vi "Save.vi"(8 "error in (no error)":errorcluster, 10 "Path":path=path "", 11 "Plot ID In":T1 format="%x") -> (0 "error out":errorcluster, 3 "Plot ID Out":T1 format="%x")   [LabVIEW 2013, in "Advanced Plotting Toolkit.lvlib"]
doc: "Save the plot to disk. The format is determined by the file extension. Supported formats are PDF, PNG, BMP, TIFF, JPEG, and GIF."
uses:
  Advanced Plotting Toolkit.lvlib
  typedefs/PlotID.ctl
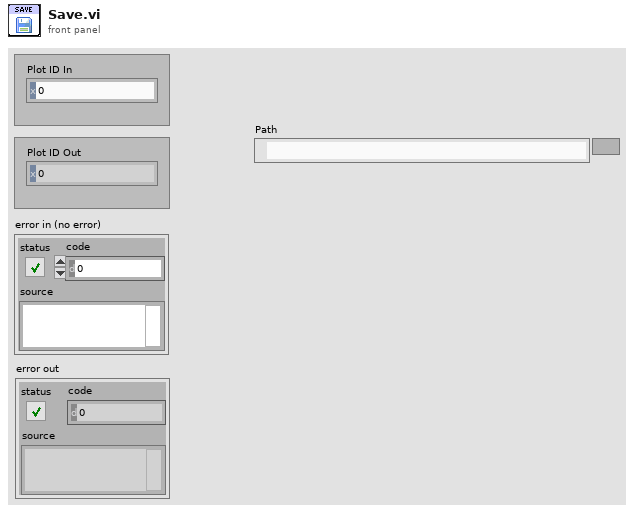
[diagram p1: front panel]
types:
  T1 = typedef "Advanced Plotting Toolkit.lvlib/PlotID.ctl" = i32
  T2 = typedef "Advanced Plotting Toolkit.lvlib/KeyValue.ctl" = cluster{"Key":string, "Value":string}
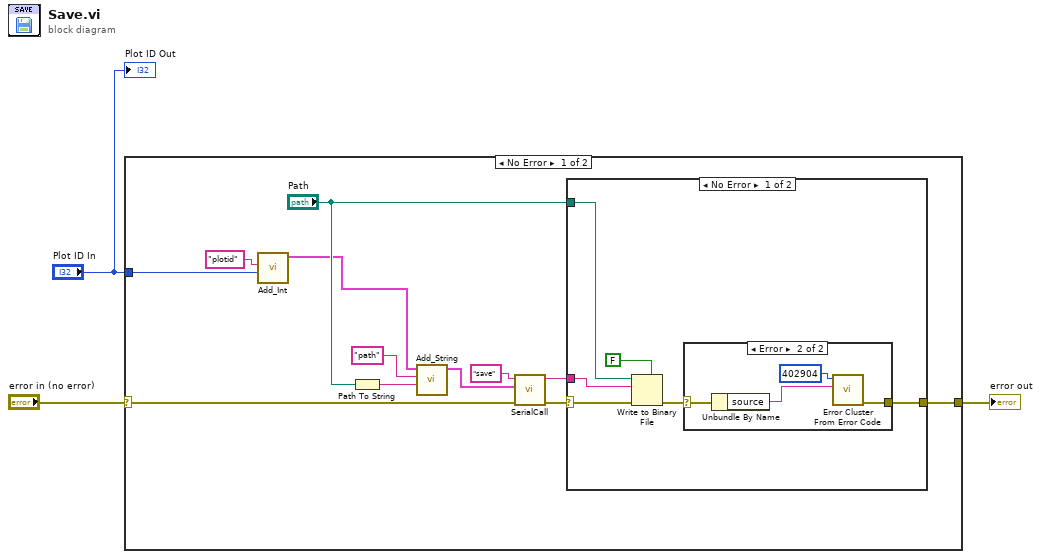
[diagram p0: block diagram]
diagram:
  n1 = case shown="No Error" "error in (no error)" {
    selector: "error in (no error)" -> [w11 w28]
    tunnel: "Plot ID In" -> [w10 _]
    tunnel: [w12 w28] -> w2
    frame No Error {
      n2 = call "Add_Int.vi"("Value"=w10, "Key"="plotid" ("Keyword")) -> ("Keyword Array Out"=w4:T2[])  [unwired: 9 in]
      n3 = Path To String(path="Path") -> (string=w7:string)
      n4 = call "Add_String.vi"("Value"=w7, "Key"="path", "Keyword Array"=w4) -> ("Keyword Array Out"=w8:T2[])  [unwired: 8 in]
      n5 = call "SerialCall.vi"("error in (no error)"=w11, "data"=w8, "Resource"="save") -> ("error out"=w13:errorcluster, "Response"=w9:string)  [unwired: 7 in]
      n6 = case shown="No Error" w13 {
        selector: w13 -> [w20 w27]
        tunnel: w9 -> [w21 _]
        tunnel: [w16 w27] -> w12
        tunnel: "Path" -> [w18 _]
        frame No Error {
          n7 = Write to Binary File(file (use dialog)=w18, data=w21, error in=w20, 5:FALSE ("prepend array or string size? (T)")) -> (error out=w17:errorcluster)  [unwired: 2 in, 2 out]
          n8 = case shown="Error" w17 {
            selector: w17 -> [w22 w25]
            tunnel: [w22 w23] -> w16
            frame No Error {
            }
            frame Error {
              n9 = Unbundle By Name(w25) -> ("source"=w24:string)
              n10 = call <vilib>:"Error Cluster From Error Code.vi"("error message (\"\")"=w24, "error code (0)"=402904) -> ("error out"=w23:errorcluster)  [unwired: 7 in]
            }
          }
        }
        frame Error {
        }
      }
    }
    frame Error {
    }
  }
  "error out" <- w2
  "Plot ID Out" <- "Plot ID In"
